vi "PrErrorSubVI.vi"(3 "eb/n0":cdb) -> (9 "Amplitude":dbl=10.0 format="%0.2p")   [LabVIEW 2019]
uses:
  <vilib>/imath/engines/lvmath2/RunTimeEngine/NodeEndStatement/NIMS_NodeEndStatement_Output.vi
  <instcachedir>/0/NIMS_NodeEndStatement_Output_53EC0D466D134D7ABD903AC30B43404B.lvgen/NIMS_NodeEndStatement_Output_53EC0D466D134D7ABD903AC30B43404B_009.vi
  <vilib>/imath/engines/lvmath2/RunTimeEngine/ErrorHandling/NIMS_Finalize Error.vi
panel:
  in  "sigma_in":dbl
  in  "s":dbl
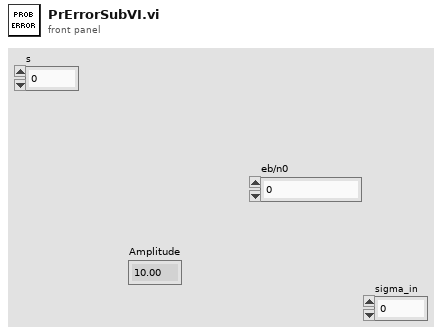
[diagram p1: front panel]
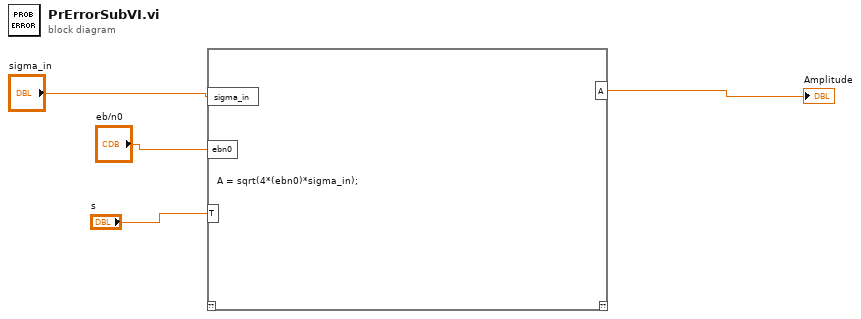
[diagram p0: block diagram]
diagram:
  n1 = mathscript code="A = sqrt(4*(ebn0)*sigma_in);"("T"="s", "ebn0"="eb/n0", "sigma_in"="sigma_in") -> ("A"=→"Amplitude":cdb)  [unwired: 1 in, 1 out]
